vi "Speed From FFT (RT).vi"() -> ()   [LabVIEW 2013]
uses:
  <vilib>/Utility/file.llb/Read From Spreadsheet File (DBL).vi
  <vilib>/FPGAPlugInAG/sbRIO-9626/niLvFpga_Open_sbRIO-9626.vi
  <vilib>/rvi/interface/common/dynamic/niFpgaDynamicAddResources.vi
  <vilib>/FPGAPlugInAG/Dynamic/niLvFpga_Abort_Dynamic.vi
  <vilib>/FPGAPlugInAG/Dynamic/niLvFpga_Run_Dynamic.vi
  <vilib>/rvi/interface/common/niFpgaWaitOnOcc.vi
  <vilib>/Utility/error.llb/Error Cluster From Error Code.vi
  <vilib>/rvi/errors/niLvFpgaAdjustHostInterfaceError.vi
  <vilib>/rvi/interface/nirviOpenFPGA/nirviOpenFPGA.xnode
  FPGA Bitfiles/SpeedFromFFT.lvbitx
  <vilib>/rvi/interface/nirviMethod/nirviMethod.xnode
  <vilib>/rvi/interface/nirviReadWriteControl/nirviReadWriteControl.xnode
  <vilib>/FPGAPlugInAG/Dynamic/niLvFpga_StartFifo_Dynamic.vi
  <vilib>/rvi/errors/niLvFpgaMergeErrorWithErrorCode.vi
  <vilib>/FPGAPlugInAG/Dynamic/niLvFpga_ReadFifo_Dynamic.vi
  <vilib>/FPGAPlugInAG/Dynamic/niLvFpga_WriteFifo_Dynamic.vi
  NiFpgaLv.dll
  <vilib>/rvi/interface/Simulation/niFpgaSimulationCallBeginRW.vi
panel:
  out "Loop Started?":bool
  out "Empty Elements Remaining":u32
  out "Timeout? FFTval Ever":bool
  out "Timeout? FFTval":bool
  out "Timeout? D2R Ever":bool
  out "Timeout? D2R":bool
  out "Setup Error?":bool
  in  "stop":bool
  out "error out":errorcluster
  out "Array":fxp<+,16,4>[](array[numeric])
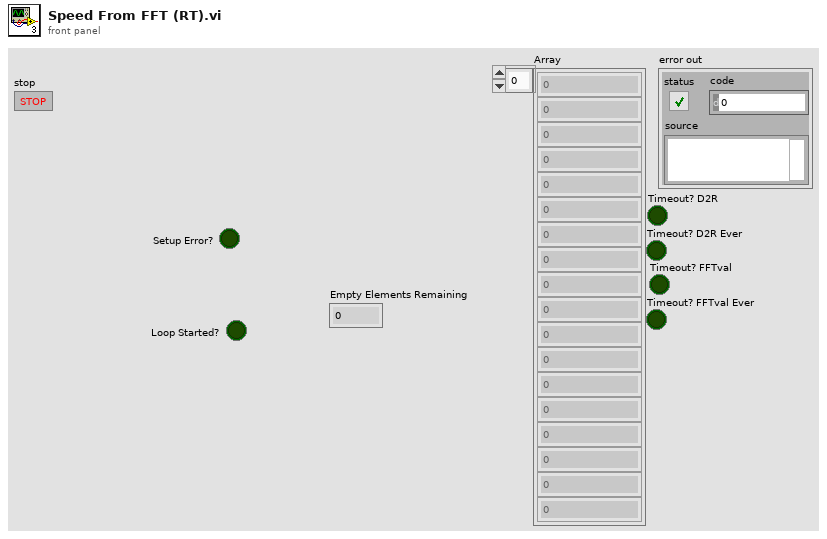
[diagram p1: front panel]
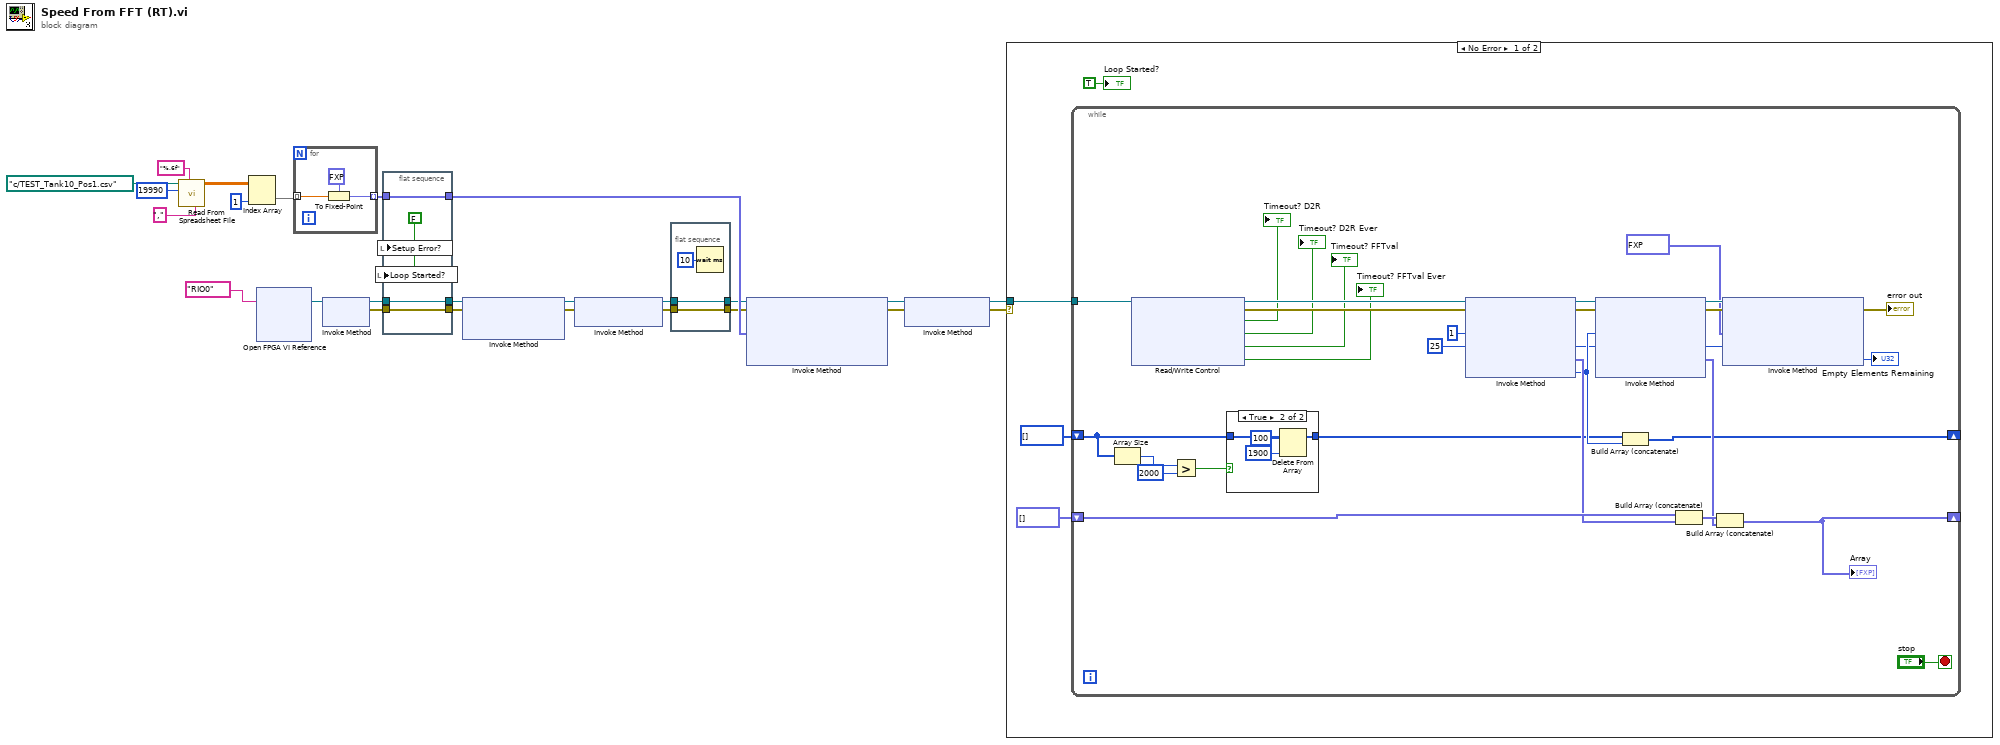
[diagram p0: block diagram]
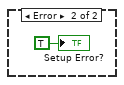
[diagram p3: hidden frame]
diagram:
  n1 = call-poly <vilib>:"Read From Spreadsheet File.vi"("delimiter (\\t)"="," ("delimiter (\\t)"), "format (%.3f)"="%.6f", "number of rows (all:-1)"=19990, "file path (dialog if empty)"=path "c:/TEST_Tank10_Pos1.csv") -> ("all rows"=w20:dbl[][])  [unwired: 3 in, 4 out]
  n2 = Index Array(array=w20, index (col)=1 ("disabled index (col)")) -> (element=w18:dbl[])  [unwired: 1 in]
  n3 = xnode "Open FPGA VI Reference"("resource name"=tag "RIO0") -> ("FPGA VI Reference Out"=w1:refnum<k20>)  [unwired: 1 in, 1 out]
  n4 = for {
    tunnel: w18 -> [w28] mode=indexing
    tunnel: [w26] -> w17 mode=indexing
    n5 = To Fixed-Point(fixed-point type=fxp<+,16,4> 0.0, number=w28) -> (fixed-point=w26:fxp<+,16,4>)
  }
  n6 = xnode "Invoke Method"("FPGA VI Reference In"=w1) -> ("FPGA VI Reference Out"=w14:refnum<k20>, "error out"=w12:errorcluster)  [unwired: 1 in]
  n7 = flat-sequence {
    tunnel: w17 -> [w32]
    tunnel: [w32] -> w9
    tunnel: w14 -> [w31]
    tunnel: [w31] -> w13
    tunnel: w12 -> [w30]
    tunnel: [w30] -> w11
    frame #0 {
      w29 = FALSE ("Setup Error?")
      n8 = local write "Loop Started?"(w29) -> ()
      n9 = local write "Setup Error?"(w29) -> ()
    }
  }
  n10 = xnode "Invoke Method"("FPGA VI Reference In"=w13, "error in"=w11) -> ("FPGA VI Reference Out"=w25:refnum<k20>, "error out"=w16:errorcluster)  [unwired: 1 in]
  n11 = xnode "Invoke Method"("FPGA VI Reference In"=w25, "error in"=w16) -> ("FPGA VI Reference Out"=w7:refnum<k20>, "error out"=w8:errorcluster)
  n12 = flat-sequence {
    tunnel: w8 -> [w33]
    tunnel: w7 -> [w34]
    tunnel: [w34] -> w6
    tunnel: [w33] -> w5
    frame #0 {
      n13 = Wait (ms)(milliseconds to wait=u32 10) -> ()  [unwired: 1 out]
    }
  }
  n14 = xnode "Invoke Method"("FPGA VI Reference In"=w6, "error in"=w5, "Data"=w9) -> ("FPGA VI Reference Out"=w4:refnum<k20>, "error out"=w3:errorcluster)  [unwired: 1 in, 1 out]
  n15 = xnode "Invoke Method"("FPGA VI Reference In"=w4, "error in"=w3) -> ("FPGA VI Reference Out"=w24:refnum<k20>, "error out"=w2:errorcluster)
  n16 = case shown="No Error" w2 {
    tunnel: w24 -> [w39 _]
    frame No Error {
      n17 = while {
        tunnel: w39 -> [w52]
        shift-right: [w56] -> _
        shift-left: fxp<+,16,4>[] [] -> [w68]
        shift-right: [w63] -> _
        shift-left: u32[] [] -> [w58]
        stop <- "stop" stop-if-true
        w42 = 25 ("Timeout (ms)")
        n18 = Array Size(array=w58) -> (size(s)=w61:i32)
        n19 = xnode "Read/Write Control"("FPGA VI Reference In"=w52) -> ("FPGA VI Reference Out"=w51:refnum<k20>, "error out"=w50:errorcluster, "Timeout? D2R"=→"Timeout? D2R":bool, "Timeout? D2R Ever"=→"Timeout? D2R Ever":bool, "Timeout? FFTval"=→"Timeout? FFTval":bool, "Timeout? FFTval Ever"=→"Timeout? FFTval Ever":bool)  [unwired: 1 in]
        n20 = Greater?(x=w61, y=2000) -> (0:w59:bool)
        n21 = case shown="True" w59 {
          tunnel: w58 -> [w69 w73]
          tunnel: [w69 w72] -> w57
          frame False {
          }
          frame True {
            n22 = Delete From Array(array=w73, length=100, index=1900) -> (array with subset deleted=w72:u32[])  [unwired: 1 out]
          }
        }
        n23 = xnode "Invoke Method"("FPGA VI Reference In"=w51, "error in"=w50, "Number of Elements"=u32 1, "Timeout (ms)"=w42) -> ("FPGA VI Reference Out"=w54:refnum<k20>, "error out"=w53:errorcluster, "Data"=w66:fxp<+,16,4>[], "Elements Remaining"=w64:u32)
        n24 = xnode "Invoke Method"("FPGA VI Reference In"=w54, "error in"=w53, "Number of Elements"=w64, "Timeout (ms)"=w42) -> ("FPGA VI Reference Out"=w45:refnum<k20>, "error out"=w44:errorcluster, "Data"=w65:fxp<+,16,4>[])  [unwired: 1 out]
        n25 = Build Array (concatenate)(w57, w64) -> (w63:u32[])
        n26 = Build Array (concatenate)(w68, w66) -> (w67:fxp<+,16,4>[])
        n27 = Build Array (concatenate)(w67, w65) -> (w56:fxp<+,16,4>[])
        "Array" <- w56
        n28 = xnode "Invoke Method"("FPGA VI Reference In"=w45, "error in"=w44, "Data"=fxp<+,16,4>[] [0.0], "Timeout (ms)"=w42) -> ("error out"=→"error out":errorcluster, "Empty Elements Remaining"=→"Empty Elements Remaining":u32)  [unwired: 1 out]
      }
      "Loop Started?" <- TRUE ("Loop Started?")
    }
    frame Error {
      "Setup Error?" <- TRUE ("Setup Error?")
    }
  }
